vi "Lab Panel V5.27.vi"() -> ()   [LabVIEW 2013] (continued)
                                }
                                frame "CYCLE TEST" {
                                }
                                frame "T-RISE TEST" {
                                }
                                }
                                n846 = Unbundle(w1488) -> ("DESCRIPTION"=w1487:string)  [unwired: 4 out]
                                n847 = Concatenate Strings(w1483, "\\", w1481, w1479, w1480, w1479) -> (w1490:string)
                                n848 = String To Path(string=w1490) -> (path=w1492:path)
                                n849 = Concatenate Strings(w1490, w1489, w1487, "-", w1486, ".tdms") -> (w1478:string)
                                n850 = Create Folder(path (use dialog)=w1492) -> (error out=w1491:errorcluster)  [unwired: 2 in, 2 out]
                                n851 = global write "Global 1.vi" "LAB03-2 FILE"(w1478) -> ()
                                n852 = call <vilib>:"Clear Errors.vi"("error in (no error)"=w1491) -> ()  [unwired: 6 in, 1 out]
                              }
                              frame #1 {
                                (unwired) FALSE
                                n853 = String To Path(string=w1502) -> (path=w1498:path)
                                n854 = TDMS Open(6:FALSE, 10:T21."create or replace" ("operation (0:open)"), 11:w1498) -> (0:w1497:errorcluster, 3:→"TDMS LAB03-2":refnum<k34>)  [unwired: 4 in]
                              }
                              frame #2 {
                                n855 = local read "SET LAB03-2"() -> (w1508:T5)
                                n856 = local read "TDMS LAB03-2"() -> (w1519:refnum<k34>)
                                n857 = Build Array("Testers Name", "Description", "Set Test Cycles", "T-Rise minutes", "T-Rise Deg C") -> (w1509:string[])
                                n858 = Unbundle(w1508) -> ("NAME"=w1507:string, "DESCRIPTION"=w1506:string, "CYCLES"=w1505:dbl, "T-RISE mins"=w1504:dbl, "T-RISE deg C"=w1503:dbl)
                                n859 = Number To Decimal String(number=w1505) -> (decimal integer string=w1518:string)  [unwired: 1 in]
                                n860 = Number To Decimal String(number=w1504) -> (decimal integer string=w1517:string)  [unwired: 1 in]
                                n861 = Number To Decimal String(number=w1503) -> (decimal integer string=w1516:string)  [unwired: 1 in]
                                n862 = Build Array(w1507, w1506, w1518, w1517, w1516) -> (w1515:string[])
                                n863 = TDMS Set Properties(5:w1515, 7:w1509, 11:w1519) -> ()  [unwired: 3 in, 4 out]
                              }
                              frame #3 {
                                n864 = local read "DISP LAB03-2"() -> (w1524:T4)
                                n865 = Concatenate Strings("LAB03-2  ", w1523) -> (w1525:string)
                                n866 = Two Button Dialog(message=w1525, 1:w1521, 2:w1522) -> (T button?=w1527:bool)
                                n867 = case shown="True" w1527 {
                                tunnel: w1524 -> [w1534 w1535]
                                tunnel: [w1534 w1535] -> w1531
                                tunnel: [w1533 w1536] -> w1530
                                tunnel: [w1532 w1536] -> w1529
                                frame False {
                                n868 = Unbundle(w1534) -> ("CYCLE"=w1533:dbl, "MINS"=w1532:dbl)  [unwired: 1 out]
                                }
                                frame True {
                                w1536 = 0.0
                                }
                                }
                                n869 = Bundle(cluster=w1531, "CYCLE"=w1530, "MINS"=w1529, "STATUS"="RUN") -> (w1520:T4)
                                n870 = local write "DISP LAB03-2"(w1520) -> ()
                              }
                              frame #4 {
                                n871 = local read "TEMP START LAB03-2"() -> (w1539:cluster{"TL":dbl, "TN":dbl})
                                n872 = Bundle(cluster=w1539, "TL"=w1537, "TN"=w1537) -> (w1538:cluster{"TL":dbl, "TN":dbl})
                                n873 = local write "TEMP START LAB03-2"(w1538) -> ()
                              }
                            }
                          }
                        }
                      }
                    }
                  }
                }
              }
              event "RUN LAB04-1": Value Change {
                n874 = event-data() -> ("NewVal"=w1544:bool)  [unwired: 1 in, 5 out]
                n875 = local write "run lab04-1"(w1544) -> ()
                n876 = case shown="True" w1544 {
                  tunnel: w1550 -> [_ w1588]
                  tunnel: w1549 -> [_ w1587]
                  tunnel: w1547 -> [w1552 w1586]
                  tunnel: w1548 -> [_ w1585]
                  tunnel: w1546 -> [_ w1584]
                  tunnel: [w1551 w1583] -> w1545
                  tunnel: w1543 -> [_ w1582]
                  tunnel: w1542 -> [_ w1581]
                  tunnel: w1541 -> [_ w1580]
                  tunnel: w1540 -> [_ w1578]
                  frame False {
                    # "stop test"
                    n877 = stacked-sequence {
                      tunnel: w1552 -> [w1561 _]
                      tunnel: [w1553 _] -> w1551
                      frame #0 {
                        n878 = local read "DISP LAB04-1"() -> (w1560:T4)
                        n879 = Unbundle(w1560) -> ("CYCLE"=w1558:dbl, "MINS"=w1559:dbl)  [unwired: 1 out]
                        n880 = case shown="\"CYCLE TEST\"" w1561 {
                          tunnel: w1559 -> [_ _ w1568]
                          tunnel: w1558 -> [w1566 w1567 _]
                          tunnel: [w1566 w1567 w1568] -> w1557
                          frame "CHART TEST", Default {
                          }
                          frame "CYCLE TEST" {
                          }
                          frame "T-RISE TEST" {
                          }
                        }
                        n881 = local read "TDMS LAB04-1"() -> (w1565:refnum<k34>)
                        n882 = Build Array("STOPPED") -> (w1562:string[])
                        n883 = Build Array(w1557) -> (w1556:dbl[])
                        n884 = TDMS Write(0:w1565, 5:"TEST RESULT", 7:w1562, 9:w1556) -> (4:w1554:refnum<k34>, 15:w1555:errorcluster)  [unwired: 2 in, 2 out]
                        n885 = TDMS Close(8:w1555, 11:w1554) -> (0:w1553:errorcluster)  [unwired: 1 out]
                      }
                      frame #1 {
                        n886 = local read "DISP LAB04-1"() -> (w1572:T4)
                        n887 = stacked-sequence {
                          tunnel: "LAB04-1" -> [w1574 w1576]
                          frame #0 {
                            n888 = call "sub vi - defrag tdms v1.vi"("panel id"=w1574) -> ("error out"=w1573:errorcluster)  [unwired: 10 in]
                            n889 = local write "data file error"(w1573) -> ()
                          }
                          frame #1 {
                            n890 = call "Save data file (stop) v3.vi"("panel id"=w1576) -> ("network file save error"=w1575:errorcluster)  [unwired: 9 in, 1 out]
                            n891 = local write "RESULT LAB04-1"(FALSE) -> ()
                            n892 = local write "data file error"(w1575) -> ()
                          }
                        }
                        n893 = Bundle(cluster=w1572, "STATUS"="STOP") -> (w1570:T4)  [unwired: 2 in]
                        n894 = local write "DISP LAB04-1"(w1570) -> ()
                      }
                    }
                  }
                  frame True {
                    n895 = local read "SIG LAB04-1"() -> (w1579:T2)
                    n896 = stacked-sequence {
                      seq-local: [w1590 _] -> [_ w1594]
                      tunnel: w1588 -> [_ w1604]
                      tunnel: w1587 -> [_ w1603]
                      tunnel: w1586 -> [_ w1602]
                      tunnel: w1585 -> [_ w1601]
                      tunnel: w1584 -> [_ w1600]
                      tunnel: [_ w1599] -> w1583
                      tunnel: w1582 -> [_ w1598]
                      tunnel: w1581 -> [_ w1597]
                      tunnel: w1580 -> [_ w1596]
                      tunnel: w1579 -> [w1589 w1595]
                      tunnel: w1578 -> [_ w1593]
                      frame #0 {
                        n897 = Unbundle(w1589) -> ("AMPS"=w1592:dbl)  [unwired: 4 out]
                        n898 = call "Check For Amps on v1.vi"("ID"="LAB04-1", "amps"=w1592) -> ("amps"=w1590:bool)  [unwired: 9 in]
                      }
                      frame #1 {
                        n899 = case shown="True" w1594 {
                          tunnel: w1604 -> [_ w1617]
                          tunnel: w1603 -> [_ w1616]
                          tunnel: w1602 -> [_ w1615]
                          tunnel: w1601 -> [_ w1614]
                          tunnel: w1600 -> [_ w1613]
                          tunnel: [errorcluster {"status"=FALSE, "code"=0, "source"=""} ("error out") w1612] -> w1599
                          tunnel: w1598 -> [_ w1611]
                          tunnel: w1597 -> [_ w1610]
                          tunnel: w1596 -> [_ w1609]
                          tunnel: w1595 -> [_ w1608]
                          tunnel: w1593 -> [_ w1607]
                          frame False {
                            w1605 = FALSE
                            n900 = local write "RUN LAB04-1"(w1605) -> ()
                            n901 = local write "run lab04-1"(w1605) -> ()
                          }
                          frame True {
                            n902 = stacked-sequence {
                              seq-local: [w1618 _ _ _ _] -> [_ w1642 _ _ _]
                              tunnel: w1617 -> [w1623 _ _ _ _]
                              tunnel: w1616 -> [w1619 _ _ _ _]
                              tunnel: w1615 -> [w1633 _ _ _ _]
                              tunnel: w1614 -> [w1626 _ _ _ _]
                              tunnel: w1613 -> [w1621 _ _ _ _]
                              tunnel: [_ w1637 _ _ _] -> w1612
                              tunnel: w1611 -> [_ _ _ w1663 _]
                              tunnel: w1610 -> [_ _ _ w1662 _]
                              tunnel: w1609 -> [_ _ _ w1661 _]
                              tunnel: w1608 -> [_ _ _ _ _]
                              tunnel: w1607 -> [_ _ _ _ w1677]
                              frame #0 {
                                w1620 = "\\"
                                n903 = local read "SET LAB04-1"() -> (w1628:T5)
                                n904 = case shown="\"CYCLE TEST\"" w1633 {
                                tunnel: ["L04-1-CHART TEST-" "L04-1-CYCLE TEST-" "L04-1-T-RISE TEST-"] -> w1629
                                frame "CHART TEST", Default {
                                }
                                frame "CYCLE TEST" {
                                }
                                frame "T-RISE TEST" {
                                }
                                }
                                n905 = Unbundle(w1628) -> ("DESCRIPTION"=w1627:string)  [unwired: 4 out]
                                n906 = Concatenate Strings(w1623, "\\", w1621, w1620, w1619, w1620) -> (w1630:string)
                                n907 = String To Path(string=w1630) -> (path=w1632:path)
                                n908 = Concatenate Strings(w1630, w1629, w1627, "-", w1626, ".tdms") -> (w1618:string)
                                n909 = Create Folder(path (use dialog)=w1632) -> (error out=w1631:errorcluster)  [unwired: 2 in, 2 out]
                                n910 = global write "Global 1.vi" "LAB04-1 FILE"(w1618) -> ()
                                n911 = call <vilib>:"Clear Errors.vi"("error in (no error)"=w1631) -> ()  [unwired: 6 in, 1 out]
                              }
                              frame #1 {
                                (unwired) FALSE
                                n912 = String To Path(string=w1642) -> (path=w1638:path)
                                n913 = TDMS Open(6:FALSE, 10:T21."create or replace" ("operation (0:open)"), 11:w1638) -> (0:w1637:errorcluster, 3:→"TDMS LAB04-1":refnum<k34>)  [unwired: 4 in]
                              }
                              frame #2 {
                                n914 = local read "SET LAB04-1"() -> (w1648:T5)
                                n915 = local read "TDMS LAB04-1"() -> (w1659:refnum<k34>)
                                n916 = Build Array("Testers Name", "Description", "Set Test Cycles", "T-Rise minutes", "T-Rise Deg C") -> (w1649:string[])
                                n917 = Unbundle(w1648) -> ("NAME"=w1647:string, "DESCRIPTION"=w1646:string, "CYCLES"=w1645:dbl, "T-RISE mins"=w1644:dbl, "T-RISE deg C"=w1643:dbl)
                                n918 = Number To Decimal String(number=w1645) -> (decimal integer string=w1658:string)  [unwired: 1 in]
                                n919 = Number To Decimal String(number=w1644) -> (decimal integer string=w1657:string)  [unwired: 1 in]
                                n920 = Number To Decimal String(number=w1643) -> (decimal integer string=w1656:string)  [unwired: 1 in]
                                n921 = Build Array(w1647, w1646, w1658, w1657, w1656) -> (w1655:string[])
                                n922 = TDMS Set Properties(5:w1655, 7:w1649, 11:w1659) -> ()  [unwired: 3 in, 4 out]
                              }
                              frame #3 {
                                n923 = local read "DISP LAB04-1"() -> (w1664:T4)
                                n924 = Concatenate Strings("LAB04-1  ", w1663) -> (w1665:string)
                                n925 = Two Button Dialog(message=w1665, 1:w1661, 2:w1662) -> (T button?=w1667:bool)
                                n926 = case shown="True" w1667 {
                                tunnel: w1664 -> [w1674 w1675]
                                tunnel: [w1674 w1675] -> w1671
                                tunnel: [w1673 w1676] -> w1670
                                tunnel: [w1672 w1676] -> w1669
                                frame False {
                                n927 = Unbundle(w1674) -> ("CYCLE"=w1673:dbl, "MINS"=w1672:dbl)  [unwired: 1 out]
                                }
                                frame True {
                                w1676 = 0.0
                                }
                                }
                                n928 = Bundle(cluster=w1671, "CYCLE"=w1670, "MINS"=w1669, "STATUS"="RUN") -> (w1660:T4)
                                n929 = local write "DISP LAB04-1"(w1660) -> ()
                              }
                              frame #4 {
                                n930 = local read "TEMP START LAB04-1"() -> (w1679:cluster{"TL":dbl, "TN":dbl})
                                n931 = Bundle(cluster=w1679, "TL"=w1677, "TN"=w1677) -> (w1678:cluster{"TL":dbl, "TN":dbl})
                                n932 = local write "TEMP START LAB04-1"(w1678) -> ()
                              }
                            }
                          }
                        }
                      }
                    }
                  }
                }
              }
              event "RUN LAB04-2": Value Change {
                n933 = event-data() -> ("NewVal"=w1684:bool)  [unwired: 1 in, 5 out]
                n934 = local write "run lab04-2"(w1684) -> ()
                n935 = case shown="True" w1684 {
                  tunnel: w1690 -> [_ w1728]
                  tunnel: w1689 -> [_ w1727]
                  tunnel: w1687 -> [w1692 w1726]
                  tunnel: w1688 -> [_ w1725]
                  tunnel: w1686 -> [_ w1724]
                  tunnel: [w1691 w1723] -> w1685
                  tunnel: w1683 -> [_ w1722]
                  tunnel: w1682 -> [_ w1721]
                  tunnel: w1681 -> [_ w1720]
                  tunnel: w1680 -> [_ w1718]
                  frame False {
                    # "stop test"
                    n936 = stacked-sequence {
                      tunnel: w1692 -> [w1701 _]
                      tunnel: [w1693 _] -> w1691
                      frame #0 {
                        n937 = local read "DISP LAB04-2"() -> (w1700:T4)
                        n938 = Unbundle(w1700) -> ("CYCLE"=w1698:dbl, "MINS"=w1699:dbl)  [unwired: 1 out]
                        n939 = case shown="\"CYCLE TEST\"" w1701 {
                          tunnel: w1699 -> [_ _ w1708]
                          tunnel: w1698 -> [w1706 w1707 _]
                          tunnel: [w1706 w1707 w1708] -> w1697
                          frame "CHART TEST", Default {
                          }
                          frame "CYCLE TEST" {
                          }
                          frame "T-RISE TEST" {
                          }
                        }
                        n940 = local read "TDMS LAB04-2"() -> (w1705:refnum<k34>)
                        n941 = Build Array("STOPPED") -> (w1702:string[])
                        n942 = Build Array(w1697) -> (w1696:dbl[])
                        n943 = TDMS Write(0:w1705, 5:"TEST RESULT", 7:w1702, 9:w1696) -> (4:w1694:refnum<k34>, 15:w1695:errorcluster)  [unwired: 2 in, 2 out]
                        n944 = TDMS Close(8:w1695, 11:w1694) -> (0:w1693:errorcluster)  [unwired: 1 out]
                      }
                      frame #1 {
                        n945 = local read "DISP LAB04-2"() -> (w1712:T4)
                        n946 = stacked-sequence {
                          tunnel: "LAB04-2" -> [w1714 w1716]
                          frame #0 {
                            n947 = call "sub vi - defrag tdms v1.vi"("panel id"=w1714) -> ("error out"=w1713:errorcluster)  [unwired: 10 in]
                            n948 = local write "data file error"(w1713) -> ()
                          }
                          frame #1 {
                            n949 = call "Save data file (stop) v3.vi"("panel id"=w1716) -> ("network file save error"=w1715:errorcluster)  [unwired: 9 in, 1 out]
                            n950 = local write "RESULT LAB04-2"(FALSE) -> ()
                            n951 = local write "data file error"(w1715) -> ()
                          }
                        }
                        n952 = Bundle(cluster=w1712, "STATUS"="STOP") -> (w1710:T4)  [unwired: 2 in]
                        n953 = local write "DISP LAB04-2"(w1710) -> ()
                      }
                    }
                  }
                  frame True {
                    n954 = local read "SIG LAB04-2"() -> (w1719:T2)
                    n955 = stacked-sequence {
                      seq-local: [w1730 _] -> [_ w1734]
                      tunnel: w1728 -> [_ w1744]
                      tunnel: w1727 -> [_ w1743]
                      tunnel: w1726 -> [_ w1742]
                      tunnel: w1725 -> [_ w1741]
                      tunnel: w1724 -> [_ w1740]
                      tunnel: [_ w1739] -> w1723
                      tunnel: w1722 -> [_ w1738]
                      tunnel: w1721 -> [_ w1737]
                      tunnel: w1720 -> [_ w1736]
                      tunnel: w1719 -> [w1729 w1735]
                      tunnel: w1718 -> [_ w1733]
                      frame #0 {
                        n956 = Unbundle(w1729) -> ("AMPS"=w1732:dbl)  [unwired: 4 out]
                        n957 = call "Check For Amps on v1.vi"("ID"="LAB04-2", "amps"=w1732) -> ("amps"=w1730:bool)  [unwired: 9 in]
                      }
                      frame #1 {
                        n958 = case shown="True" w1734 {
                          tunnel: w1744 -> [_ w1757]
                          tunnel: w1743 -> [_ w1756]
                          tunnel: w1742 -> [_ w1755]
                          tunnel: w1741 -> [_ w1754]
                          tunnel: w1740 -> [_ w1753]
                          tunnel: [errorcluster {"status"=FALSE, "code"=0, "source"=""} ("error out") w1752] -> w1739
                          tunnel: w1738 -> [_ w1751]
                          tunnel: w1737 -> [_ w1750]
                          tunnel: w1736 -> [_ w1749]
                          tunnel: w1735 -> [_ w1748]
                          tunnel: w1733 -> [_ w1747]
                          frame False {
                            w1745 = FALSE
                            n959 = local write "RUN LAB04-2"(w1745) -> ()
                            n960 = local write "run lab04-2"(w1745) -> ()
                          }
                          frame True {
                            n961 = stacked-sequence {
                              seq-local: [w1758 _ _ _ _] -> [_ w1782 _ _ _]
                              tunnel: w1757 -> [w1763 _ _ _ _]
                              tunnel: w1756 -> [w1759 _ _ _ _]
                              tunnel: w1755 -> [w1773 _ _ _ _]
                              tunnel: w1754 -> [w1766 _ _ _ _]
                              tunnel: w1753 -> [w1761 _ _ _ _]
                              tunnel: [_ w1777 _ _ _] -> w1752
                              tunnel: w1751 -> [_ _ _ w1803 _]
                              tunnel: w1750 -> [_ _ _ w1802 _]
                              tunnel: w1749 -> [_ _ _ w1801 _]
                              tunnel: w1748 -> [_ _ _ _ _]
                              tunnel: w1747 -> [_ _ _ _ w1817]
                              frame #0 {
                                w1760 = "\\"
                                n962 = local read "SET LAB04-2"() -> (w1768:T5)
                                n963 = case shown="\"CHART TEST\", Default" w1773 {
                                tunnel: ["L04-2-CHART TEST-" "L04-2-CYCLE TEST-" "L04-2-T-RISE TEST-"] -> w1769
                                frame "CHART TEST", Default {
                                }
                                frame "CYCLE TEST" {
                                }
                                frame "T-RISE TEST" {
                                }
                                }
                                n964 = Unbundle(w1768) -> ("DESCRIPTION"=w1767:string)  [unwired: 4 out]
                                n965 = Concatenate Strings(w1763, "\\", w1761, w1760, w1759, w1760) -> (w1770:string)
                                n966 = String To Path(string=w1770) -> (path=w1772:path)
                                n967 = Concatenate Strings(w1770, w1769, w1767, "-", w1766, ".tdms") -> (w1758:string)
                                n968 = Create Folder(path (use dialog)=w1772) -> (error out=w1771:errorcluster)  [unwired: 2 in, 2 out]
                                n969 = global write "Global 1.vi" "LAB04-2 FILE"(w1758) -> ()
                                n970 = call <vilib>:"Clear Errors.vi"("error in (no error)"=w1771) -> ()  [unwired: 6 in, 1 out]
                              }
                              frame #1 {
                                (unwired) FALSE
                                n971 = String To Path(string=w1782) -> (path=w1778:path)
                                n972 = TDMS Open(6:FALSE, 10:T21."create or replace" ("operation (0:open)"), 11:w1778) -> (0:w1777:errorcluster, 3:→"TDMS LAB04-2":refnum<k34>)  [unwired: 4 in]
                              }
                              frame #2 {
                                n973 = local read "SET LAB04-2"() -> (w1788:T5)
                                n974 = local read "TDMS LAB04-2"() -> (w1799:refnum<k34>)
                                n975 = Build Array("Testers Name", "Description", "Set Test Cycles", "T-Rise minutes", "T-Rise Deg C") -> (w1789:string[])
                                n976 = Unbundle(w1788) -> ("NAME"=w1787:string, "DESCRIPTION"=w1786:string, "CYCLES"=w1785:dbl, "T-RISE mins"=w1784:dbl, "T-RISE deg C"=w1783:dbl)
                                n977 = Number To Decimal String(number=w1785) -> (decimal integer string=w1798:string)  [unwired: 1 in]
                                n978 = Number To Decimal String(number=w1784) -> (decimal integer string=w1797:string)  [unwired: 1 in]
                                n979 = Number To Decimal String(number=w1783) -> (decimal integer string=w1796:string)  [unwired: 1 in]
                                n980 = Build Array(w1787, w1786, w1798, w1797, w1796) -> (w1795:string[])
                                n981 = TDMS Set Properties(5:w1795, 7:w1789, 11:w1799) -> ()  [unwired: 3 in, 4 out]
                              }
                              frame #3 {
                                n982 = local read "DISP LAB04-2"() -> (w1804:T4)
                                n983 = Concatenate Strings("LAB04-2 ", w1803) -> (w1805:string)
                                n984 = Two Button Dialog(message=w1805, 1:w1801, 2:w1802) -> (T button?=w1807:bool)
                                n985 = case shown="True" w1807 {
                                tunnel: w1804 -> [w1814 w1815]
                                tunnel: [w1814 w1815] -> w1811
                                tunnel: [w1813 w1816] -> w1810
                                tunnel: [w1812 w1816] -> w1809
                                frame False {
                                n986 = Unbundle(w1814) -> ("CYCLE"=w1813:dbl, "MINS"=w1812:dbl)  [unwired: 1 out]
                                }
                                frame True {
                                w1816 = 0.0
                                }
                                }
                                n987 = Bundle(cluster=w1811, "CYCLE"=w1810, "MINS"=w1809, "STATUS"="RUN") -> (w1800:T4)
                                n988 = local write "DISP LAB04-2"(w1800) -> ()
                              }
                              frame #4 {
                                n989 = local read "TEMP START LAB04-2"() -> (w1819:cluster{"TL":dbl, "TN":dbl})
                                n990 = Bundle(cluster=w1819, "TL"=w1817, "TN"=w1817) -> (w1818:cluster{"TL":dbl, "TN":dbl})
                                n991 = local write "TEMP START LAB04-2"(w1818) -> ()
                              }
                            }
                          }
                        }
                      }
                    }
                  }
                }
              }
              event "RUN LAB05-1": Value Change {
                n992 = event-data() -> ("NewVal"=w1824:bool)  [unwired: 1 in, 5 out]
                n993 = local write "run lab05-1"(w1824) -> ()
                n994 = case shown="True" w1824 {
                  tunnel: w1830 -> [_ w1868]
                  tunnel: w1829 -> [_ w1867]
                  tunnel: w1827 -> [w1832 w1866]
                  tunnel: w1828 -> [_ w1865]
                  tunnel: w1826 -> [_ w1864]
                  tunnel: [w1831 w1863] -> w1825
                  tunnel: w1823 -> [_ w1862]
                  tunnel: w1822 -> [_ w1861]
                  tunnel: w1821 -> [_ w1860]
                  tunnel: w1820 -> [_ w1858]
                  frame False {
                    # "stop test"
                    n995 = stacked-sequence {
                      tunnel: w1832 -> [w1841 _]
                      tunnel: [w1833 _] -> w1831
                      frame #0 {
                        n996 = local read "DISP LAB05-1"() -> (w1840:T4)
                        n997 = Unbundle(w1840) -> ("CYCLE"=w1838:dbl, "MINS"=w1839:dbl)  [unwired: 1 out]
                        n998 = case shown="\"CYCLE TEST\"" w1841 {
                          tunnel: w1839 -> [_ _ w1848]
                          tunnel: w1838 -> [w1846 w1847 _]
                          tunnel: [w1846 w1847 w1848] -> w1837
                          frame "CHART TEST", Default {
                          }
                          frame "CYCLE TEST" {
                          }
                          frame "T-RISE TEST" {
                          }
                        }
                        n999 = local read "TDMS LAB05-1"() -> (w1845:refnum<k34>)
                        n1000 = Build Array("STOPPED") -> (w1842:string[])
                        n1001 = Build Array(w1837) -> (w1836:dbl[])
                        n1002 = TDMS Write(0:w1845, 5:"TEST RESULT", 7:w1842, 9:w1836) -> (4:w1834:refnum<k34>, 15:w1835:errorcluster)  [unwired: 2 in, 2 out]
                        n1003 = TDMS Close(8:w1835, 11:w1834) -> (0:w1833:errorcluster)  [unwired: 1 out]
                      }
                      frame #1 {
                        n1004 = local read "DISP LAB05-1"() -> (w1852:T4)
                        n1005 = stacked-sequence {
                          tunnel: "LAB05-1" -> [w1854 w1856]
                          frame #0 {
                            n1006 = call "sub vi - defrag tdms v1.vi"("panel id"=w1854) -> ("error out"=w1853:errorcluster)  [unwired: 10 in]
                            n1007 = local write "data file error"(w1853) -> ()
                          }
                          frame #1 {
                            n1008 = call "Save data file (stop) v3.vi"("panel id"=w1856) -> ("network file save error"=w1855:errorcluster)  [unwired: 9 in, 1 out]
                            n1009 = local write "RESULT LAB05-1"(FALSE) -> ()
                            n1010 = local write "data file error"(w1855) -> ()
                          }
                        }
                        n1011 = Bundle(cluster=w1852, "STATUS"="STOP") -> (w1850:T4)  [unwired: 2 in]
                        n1012 = local write "DISP LAB05-1"(w1850) -> ()
                      }
                    }
                  }
                  frame True {
                    n1013 = local read "SIG LAB05-1"() -> (w1859:T2)
                    n1014 = stacked-sequence {
                      seq-local: [w1870 _] -> [_ w1874]
                      tunnel: w1868 -> [_ w1884]
                      tunnel: w1867 -> [_ w1883]
                      tunnel: w1866 -> [_ w1882]
                      tunnel: w1865 -> [_ w1881]
                      tunnel: w1864 -> [_ w1880]
                      tunnel: [_ w1879] -> w1863
                      tunnel: w1862 -> [_ w1878]
                      tunnel: w1861 -> [_ w1877]
                      tunnel: w1860 -> [_ w1876]
                      tunnel: w1859 -> [w1869 w1875]
                      tunnel: w1858 -> [_ w1873]
                      frame #0 {
                        n1015 = Unbundle(w1869) -> ("AMPS"=w1872:dbl)  [unwired: 4 out]
                        n1016 = call "Check For Amps on v1.vi"("ID"="LAB05-1", "amps"=w1872) -> ("amps"=w1870:bool)  [unwired: 9 in]
                      }
                      frame #1 {
                        n1017 = case shown="True" w1874 {
                          tunnel: w1884 -> [_ w1897]
                          tunnel: w1883 -> [_ w1896]
                          tunnel: w1882 -> [_ w1895]
                          tunnel: w1881 -> [_ w1894]
                          tunnel: w1880 -> [_ w1893]
                          tunnel: [errorcluster {"status"=FALSE, "code"=0, "source"=""} ("error out") w1892] -> w1879
                          tunnel: w1878 -> [_ w1891]
                          tunnel: w1877 -> [_ w1890]
                          tunnel: w1876 -> [_ w1889]
                          tunnel: w1875 -> [_ w1888]
                          tunnel: w1873 -> [_ w1887]
                          frame False {
                            w1885 = FALSE
                            n1018 = local write "RUN LAB05-1"(w1885) -> ()
                            n1019 = local write "run lab05-1"(w1885) -> ()
                          }
                          frame True {
                            n1020 = stacked-sequence {
                              seq-local: [w1898 _ _ _ _] -> [_ w1922 _ _ _]
                              tunnel: w1897 -> [w1903 _ _ _ _]
                              tunnel: w1896 -> [w1899 _ _ _ _]
                              tunnel: w1895 -> [w1913 _ _ _ _]
                              tunnel: w1894 -> [w1906 _ _ _ _]
                              tunnel: w1893 -> [w1901 _ _ _ _]
                              tunnel: [_ w1917 _ _ _] -> w1892
                              tunnel: w1891 -> [_ _ _ w1942 _]
                              tunnel: w1890 -> [_ _ _ w1941 _]
                              tunnel: w1889 -> [_ _ _ w1940 _]
                              tunnel: w1888 -> [_ _ _ _ _]
                              tunnel: w1887 -> [_ _ _ _ w1957]
                              frame #0 {
                                w1900 = "\\"
                                n1021 = local read "SET LAB05-1"() -> (w1908:T5)
                                n1022 = case shown="\"CYCLE TEST\"" w1913 {
                                tunnel: ["L05-1-CHART TEST-" "L05-1-CYCLE TEST-" "L05-1-T-RISE TEST-"] -> w1909
                                frame "CHART TEST", Default {
                                }
                                frame "CYCLE TEST" {
                                }
                                frame "T-RISE TEST" {
                                }
                                }
                                n1023 = Unbundle(w1908) -> ("DESCRIPTION"=w1907:string)  [unwired: 4 out]
                                n1024 = Concatenate Strings(w1903, "\\", w1901, w1900, w1899, w1900) -> (w1910:string)
                                n1025 = String To Path(string=w1910) -> (path=w1912:path)
                                n1026 = Concatenate Strings(w1910, w1909, w1907, "-", w1906, ".tdms") -> (w1898:string)
                                n1027 = Create Folder(path (use dialog)=w1912) -> (error out=w1911:errorcluster)  [unwired: 2 in, 2 out]
                                n1028 = global write "Global 1.vi" "LAB05-1 FILE"(w1898) -> ()
                                n1029 = call <vilib>:"Clear Errors.vi"("error in (no error)"=w1911) -> ()  [unwired: 6 in, 1 out]
                              }
                              frame #1 {
                                (unwired) FALSE
                                n1030 = String To Path(string=w1922) -> (path=w1918:path)
                                n1031 = TDMS Open(6:FALSE, 10:T21."create or replace" ("operation (0:open)"), 11:w1918) -> (0:w1917:errorcluster, 3:→"TDMS LAB05-1":refnum<k34>)  [unwired: 4 in]
                              }
                              frame #2 {
                                n1032 = local read "SET LAB05-1"() -> (w1928:T5)
                                n1033 = local read "TDMS LAB05-1"() -> (w1939:refnum<k34>)
                                n1034 = Build Array("Testers Name", "Description", "Set Test Cycles", "T-Rise minutes", "T-Rise Deg C") -> (w1929:string[])
                                n1035 = Unbundle(w1928) -> ("NAME"=w1927:string, "DESCRIPTION"=w1926:string, "CYCLES"=w1925:dbl, "T-RISE mins"=w1924:dbl, "T-RISE deg C"=w1923:dbl)
                                n1036 = Number To Decimal String(number=w1925) -> (decimal integer string=w1938:string)  [unwired: 1 in]
                                n1037 = Number To Decimal String(number=w1924) -> (decimal integer string=w1937:string)  [unwired: 1 in]
                                n1038 = Number To Decimal String(number=w1923) -> (decimal integer string=w1936:string)  [unwired: 1 in]
                                n1039 = Build Array(w1927, w1926, w1938, w1937, w1936) -> (w1935:string[])
                                n1040 = TDMS Set Properties(5:w1935, 7:w1929, 11:w1939) -> ()  [unwired: 3 in, 4 out]
                              }
                              frame #3 {
                                n1041 = local read "DISP LAB05-1"() -> (w1944:T4)
                                n1042 = Concatenate Strings("LAB05-1  ", w1942) -> (w1945:string)
                                n1043 = Two Button Dialog(message=w1945, 1:w1940, 2:w1941) -> (T button?=w1947:bool)
                                n1044 = case shown="True" w1947 {
                                tunnel: w1944 -> [w1954 w1955]
                                tunnel: [w1954 w1955] -> w1951
                                tunnel: [w1953 w1956] -> w1950
                                tunnel: [w1952 w1956] -> w1949
                                frame False {
                                n1045 = Unbundle(w1954) -> ("CYCLE"=w1953:dbl, "MINS"=w1952:dbl)  [unwired: 1 out]
                                }
                                frame True {
                                w1956 = 0.0
                                }
                                }
                                n1046 = Bundle(cluster=w1951, "CYCLE"=w1950, "MINS"=w1949, "STATUS"="RUN") -> (w1943:T4)
                                n1047 = local write "DISP LAB05-1"(w1943) -> ()
                              }
                              frame #4 {
                                n1048 = local read "TEMP START LAB05-1"() -> (w1959:cluster{"TL":dbl, "TN":dbl})
                                n1049 = Bundle(cluster=w1959, "TL"=w1957, "TN"=w1957) -> (w1958:cluster{"TL":dbl, "TN":dbl})
                                n1050 = local write "TEMP START LAB05-1"(w1958) -> ()
                              }
                            }
                          }
                        }
                      }
                    }
                  }
                }
              }
              event "RUN LAB05-2": Value Change {
                n1051 = event-data() -> ("NewVal"=w1965:bool)  [unwired: 1 in, 5 out]
                n1052 = local read "SIG LAB05-2"() -> (w1961:T2)
                n1053 = case shown="True" w1965 {
                  tunnel: w1971 -> [_ w2009]
                  tunnel: w1970 -> [_ w2008]
                  tunnel: w1968 -> [w1973 w2007]
                  tunnel: w1969 -> [_ w2006]
                  tunnel: w1967 -> [_ w2005]
                  tunnel: [w1972 w2004] -> w1966
                  tunnel: w1964 -> [_ w2003]
                  tunnel: w1963 -> [_ w2002]
                  tunnel: w1962 -> [_ w2001]
                  tunnel: w1961 -> [_ w2000]
                  tunnel: w1960 -> [_ w1999]
                  frame False {
                    # "stop test"
                    n1054 = stacked-sequence {
                      tunnel: w1973 -> [w1982 _]
                      tunnel: [w1974 _] -> w1972
                      frame #0 {
                        n1055 = local read "DISP LAB05-2"() -> (w1981:T4)
                        n1056 = Unbundle(w1981) -> ("CYCLE"=w1979:dbl, "MINS"=w1980:dbl)  [unwired: 1 out]
                        n1057 = case shown="\"CYCLE TEST\"" w1982 {
                          tunnel: w1980 -> [_ _ w1989]
                          tunnel: w1979 -> [w1987 w1988 _]
                          tunnel: [w1987 w1988 w1989] -> w1978
                          frame "CHART TEST", Default {
                          }
                          frame "CYCLE TEST" {
                          }
                          frame "T-RISE TEST" {
                          }
                        }
                        n1058 = local read "TDMS LAB05-2"() -> (w1986:refnum<k34>)
                        n1059 = Build Array("STOPPED") -> (w1983:string[])
                        n1060 = Build Array(w1978) -> (w1977:dbl[])
                        n1061 = TDMS Write(0:w1986, 5:"TEST RESULT", 7:w1983, 9:w1977) -> (4:w1975:refnum<k34>, 15:w1976:errorcluster)  [unwired: 2 in, 2 out]
                        n1062 = TDMS Close(8:w1976, 11:w1975) -> (0:w1974:errorcluster)  [unwired: 1 out]
                      }
                      frame #1 {
                        n1063 = local read "DISP LAB05-2"() -> (w1993:T4)
                        n1064 = stacked-sequence {
                          tunnel: "LAB05-2" -> [w1995 w1997]
                          frame #0 {
                            n1065 = call "sub vi - defrag tdms v1.vi"("panel id"=w1995) -> ("error out"=w1994:errorcluster)  [unwired: 10 in]
                            n1066 = local write "data file error"(w1994) -> ()
                          }
                          frame #1 {
                            n1067 = local write "RESULT LAB05-2"(FALSE) -> ()
                            n1068 = call "Save data file (stop) v3.vi"("panel id"=w1997) -> ("network file save error"=w1996:errorcluster)  [unwired: 9 in, 1 out]
                            n1069 = local write "data file error"(w1996) -> ()
                          }
                        }
                        n1070 = Bundle(cluster=w1993, "STATUS"="STOP") -> (w1991:T4)  [unwired: 2 in]
                        n1071 = local write "DISP LAB05-2"(w1991) -> ()
                      }
                    }
                  }
                  frame True {
                    n1072 = stacked-sequence {
                      seq-local: [w2011 _] -> [_ w2015]
                      tunnel: w2009 -> [_ w2025]
                      tunnel: w2008 -> [_ w2024]
                      tunnel: w2007 -> [_ w2023]
                      tunnel: w2006 -> [_ w2022]
                      tunnel: w2005 -> [_ w2021]
                      tunnel: [_ w2020] -> w2004
                      tunnel: w2003 -> [_ w2019]
                      tunnel: w2002 -> [_ w2018]
                      tunnel: w2001 -> [_ w2017]
                      tunnel: w2000 -> [w2010 w2016]
                      tunnel: w1999 -> [_ w2014]
                      frame #0 {
                        n1073 = Unbundle(w2010) -> ("AMPS"=w2013:dbl)  [unwired: 4 out]
                        n1074 = call "Check For Amps on v1.vi"("ID"="LAB05-2", "amps"=w2013) -> ("amps"=w2011:bool)  [unwired: 9 in]
                      }
                      frame #1 {
                        n1075 = case shown="True" w2015 {
                          tunnel: w2025 -> [_ w2038]
                          tunnel: w2024 -> [_ w2037]
                          tunnel: w2023 -> [_ w2036]
                          tunnel: w2022 -> [_ w2035]
                          tunnel: w2021 -> [_ w2034]
                          tunnel: [errorcluster {"status"=FALSE, "code"=0, "source"=""} ("error out") w2033] -> w2020
                          tunnel: w2019 -> [_ w2032]
                          tunnel: w2018 -> [_ w2031]
                          tunnel: w2017 -> [_ w2030]
                          tunnel: w2016 -> [_ w2029]
                          tunnel: w2014 -> [_ w2028]
                          frame False {
                            w2026 = FALSE
                            n1076 = local write "RUN LAB05-2"(w2026) -> ()
                            n1077 = local write "run lab05-2"(w2026) -> ()
                          }
                          frame True {
                            n1078 = stacked-sequence {
                              seq-local: [w2039 _ _ _ _] -> [_ w2063 _ _ _]
                              tunnel: w2038 -> [w2044 _ _ _ _]
                              tunnel: w2037 -> [w2040 _ _ _ _]
                              tunnel: w2036 -> [w2054 _ _ _ _]
                              tunnel: w2035 -> [w2047 _ _ _ _]
                              tunnel: w2034 -> [w2042 _ _ _ _]
                              tunnel: [_ w2058 _ _ _] -> w2033
                              tunnel: w2032 -> [_ _ _ w2083 _]
                              tunnel: w2031 -> [_ _ _ w2082 _]
                              tunnel: w2030 -> [_ _ _ w2081 _]
                              tunnel: w2029 -> [_ _ _ _ _]
                              tunnel: w2028 -> [_ _ _ _ w2098]
                              frame #0 {
                                w2041 = "\\"
                                n1079 = local read "SET LAB05-2"() -> (w2049:T5)
                                n1080 = case shown="\"CYCLE TEST\"" w2054 {
                                tunnel: ["L05-2-CHART TEST-" "L05-2-CYCLE TEST-" "L05-2-T-RISE TEST-"] -> w2050
                                frame "CHART TEST", Default {
                                }
                                frame "CYCLE TEST" {
                                }
                                frame "T-RISE TEST" {
                                }
                                }
                                n1081 = Unbundle(w2049) -> ("DESCRIPTION"=w2048:string)  [unwired: 4 out]
                                n1082 = Concatenate Strings(w2044, "\\", w2042, w2041, w2040, w2041) -> (w2051:string)
                                n1083 = String To Path(string=w2051) -> (path=w2053:path)
                                n1084 = Concatenate Strings(w2051, w2050, w2048, "-", w2047, ".tdms") -> (w2039:string)
                                n1085 = Create Folder(path (use dialog)=w2053) -> (error out=w2052:errorcluster)  [unwired: 2 in, 2 out]
                                n1086 = global write "Global 1.vi" "LAB05-2 FILE"(w2039) -> ()
                                n1087 = call <vilib>:"Clear Errors.vi"("error in (no error)"=w2052) -> ()  [unwired: 6 in, 1 out]
                              }
                              frame #1 {
                                (unwired) FALSE
                                n1088 = String To Path(string=w2063) -> (path=w2059:path)
                                n1089 = TDMS Open(6:FALSE, 10:T21."create or replace" ("operation (0:open)"), 11:w2059) -> (0:w2058:errorcluster, 3:→"TDMS LAB05-2":refnum<k34>)  [unwired: 4 in]
                              }
                              frame #2 {
                                n1090 = local read "SET LAB05-2"() -> (w2069:T5)
                                n1091 = local read "TDMS LAB05-2"() -> (w2080:refnum<k34>)
                                n1092 = Build Array("Testers Name", "Description", "Set Test Cycles", "T-Rise minutes", "T-Rise Deg C") -> (w2070:string[])
                                n1093 = Unbundle(w2069) -> ("NAME"=w2068:string, "DESCRIPTION"=w2067:string, "CYCLES"=w2066:dbl, "T-RISE mins"=w2065:dbl, "T-RISE deg C"=w2064:dbl)
                                n1094 = Number To Decimal String(number=w2066) -> (decimal integer string=w2079:string)  [unwired: 1 in]
                                n1095 = Number To Decimal String(number=w2065) -> (decimal integer string=w2078:string)  [unwired: 1 in]
                                n1096 = Number To Decimal String(number=w2064) -> (decimal integer string=w2077:string)  [unwired: 1 in]
                                n1097 = Build Array(w2068, w2067, w2079, w2078, w2077) -> (w2076:string[])
                                n1098 = TDMS Set Properties(5:w2076, 7:w2070, 11:w2080) -> ()  [unwired: 3 in, 4 out]
                              }
                              frame #3 {
                                n1099 = local read "DISP LAB05-2"() -> (w2085:T4)
                                n1100 = Concatenate Strings("LAB05-2  ", w2083) -> (w2086:string)
                                n1101 = Two Button Dialog(message=w2086, 1:w2081, 2:w2082) -> (T button?=w2088:bool)
                                n1102 = case shown="True" w2088 {
                                tunnel: w2085 -> [w2095 w2096]
                                tunnel: [w2095 w2096] -> w2092
                                tunnel: [w2094 w2097] -> w2091
                                tunnel: [w2093 w2097] -> w2090
                                frame False {
                                n1103 = Unbundle(w2095) -> ("CYCLE"=w2094:dbl, "MINS"=w2093:dbl)  [unwired: 1 out]
                                }
                                frame True {
                                w2097 = 0.0
                                }
                                }
                                n1104 = Bundle(cluster=w2092, "CYCLE"=w2091, "MINS"=w2090, "STATUS"="RUN") -> (w2084:T4)
                                n1105 = local write "DISP LAB05-2"(w2084) -> ()
                              }
                              frame #4 {
                                n1106 = local read "TEMP START LAB05-2"() -> (w2100:cluster{"TL":dbl, "TN":dbl})
                                n1107 = Bundle(cluster=w2100, "TL"=w2098, "TN"=w2098) -> (w2099:cluster{"TL":dbl, "TN":dbl})
                                n1108 = local write "TEMP START LAB05-2"(w2099) -> ()
                              }
                            }
                          }
                        }
                      }
                    }
                  }
                }
                n1109 = local write "run lab05-2"(w1965) -> ()
              }
            }
            n1110 = local write "data file error"(w669) -> ()
          }
          frame #5 {
            # "check if test cycles reached for cycle tests, if so then test pass"
            n1111 = stacked-sequence {
              tunnel: w2120 -> [_ _ _ _ _ _ _ _ _ _]
              tunnel: w2119 -> [_ _ _ _ _ _ _ _ _ _]
              tunnel: w2118 -> [_ _ _ _ _ _ _ _ _ _]
              tunnel: w2117 -> [_ _ _ _ _ _ _ _ _ _]
              tunnel: w2116 -> [_ _ _ _ _ _ _ _ _ _]
              tunnel: w2115 -> [_ _ _ _ _ _ _ _ _ _]
              tunnel: w2114 -> [_ _ _ _ _ _ _ _ _ _]
              tunnel: w2113 -> [_ _ _ _ _ _ _ _ _ _]
              tunnel: w2112 -> [_ _ _ _ _ _ _ _ _ _]
              tunnel: w2111 -> [_ _ _ _ _ _ _ _ _ _]
              tunnel: w2110 -> [w2126 _ _ _ _ _ _ _ _ _]
              tunnel: w2109 -> [_ w2161 _ _ _ _ _ _ _ _]
              tunnel: w2108 -> [_ _ w2201 _ _ _ _ _ _ _]
              tunnel: w2107 -> [_ _ _ w2241 _ _ _ _ _ _]
              tunnel: w2106 -> [_ _ _ _ w2281 _ _ _ _ _]
              tunnel: w2105 -> [_ _ _ _ _ w2321 _ _ _ _]
              tunnel: w2104 -> [_ _ _ _ _ _ w2361 _ _ _]
              tunnel: w2103 -> [_ _ _ _ _ _ _ w2401 _ _]
              tunnel: w2102 -> [_ _ _ _ _ _ _ _ w2441 _]
              tunnel: w2101 -> [_ _ _ _ _ _ _ _ _ w2481]
              frame #0 {
                # "LAB01-1"
                n1112 = Less?(x=w2126, y=2) -> (x < y?=w2124:bool)
                n1113 = local read "DISP LAB01-1"() -> (w2127:T4)
                n1114 = Unbundle(w2127) -> ("STATUS"=w2121:string)  [unwired: 2 out]
